vi "IMU_read_RT_streaming_data_1.0.vi"() -> ()   [LabVIEW 2016]
doc: "This example demonstrates how to stream data from the FPGA target to the host PC using DMA FIFO."
uses:
  <vilib>/userdefined/Silver/nirio_resource_slv.ctl
  <vilib>/FPGAPlugInAG/cRIO-9116/niLvFpga_Open_cRIO-9116.vi
  <vilib>/rvi/interface/common/dynamic/niFpgaDynamicAddResources.vi
  <vilib>/Utility/error.llb/Error Cluster From Error Code.vi
  <vilib>/rvi/errors/niLvFpgaAdjustHostInterfaceError.vi
  <vilib>/FPGAPlugInAG/Dynamic/niLvFpga_Close_Dynamic.vi
  <vilib>/rvi/interface/nirviOpenFPGA/nirviOpenFPGA.xnode
  FPGA Bitfiles/IMUuse_FPGATarget_IMUreadFPGAstrea_DORLY4QJmyg.lvbitx
  IMU_read_FPGA_streaming_data.vi
  <vilib>/rvi/interface/nirviReadWriteControl/nirviReadWriteControl.xnode
  <vilib>/rvi/interface/nirviMethod/nirviMethod.xnode
  <vilib>/rvi/interface/nirviCloseFPGA/nirviCloseFPGA.xnode
  <vilib>/FPGAPlugInAG/Dynamic/niLvFpga_ReadFifo_Dynamic.vi
  <vilib>/rvi/errors/niLvFpgaMergeErrorWithErrorCode.vi
  NiFpgaLv.dll
  <vilib>/rvi/interface/Simulation/niFpgaSimulationCallBeginRW.vi
panel:
  out "Angle (degree)":cluster{ext, ext, ext}(graph)
  out "Angular Rate (degree/s)":cluster{ext, ext, ext}(graph)
  in  "停止按钮":bool
  in  "波特率":T1(ring)=enum."460.8 kbps"
  in  "RIO Device":T2="RIO0"
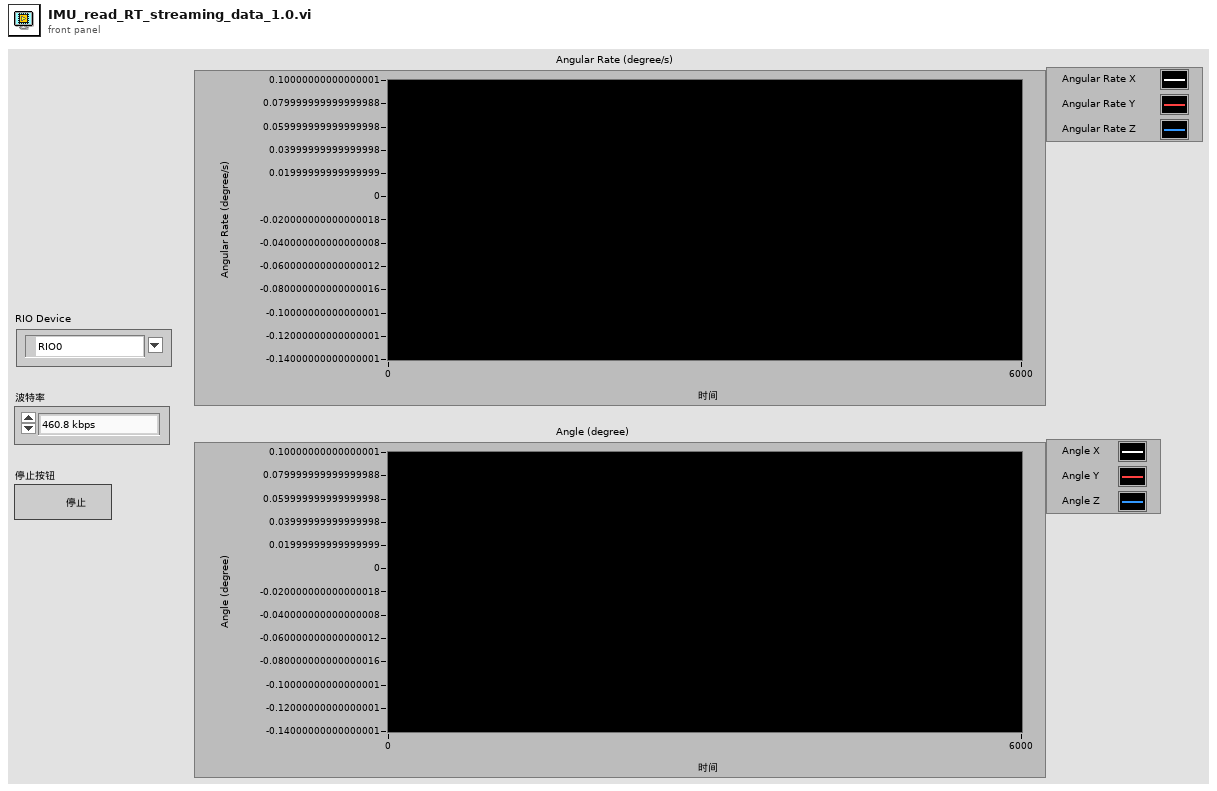
[diagram p1: front panel]
types:
  T1 = enum16{"75 bps", "110 bps", "134 bps", "150 bps", "300 bps", "600 bps", "1200 bps", "1800 bps", "2400 bps", "4800 bps", "7200 bps", "9600 bps", "14.4 kbps", "19.2 kbps", "28.8 kbps", "38.4 kbps", "57.6 kbps", "115.2 kbps", "230.4 kbps", "460.8 kbps", "921.6 kbps"}
  T2 = typedef "nirio_resource_slv.ctl" = tag
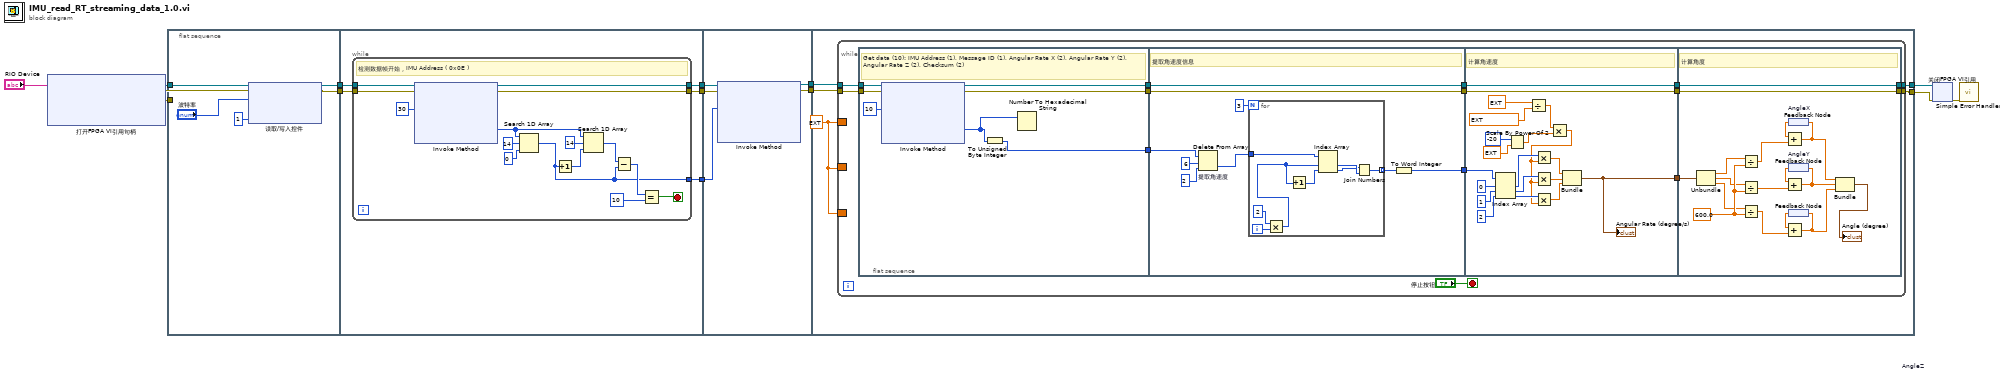
[diagram p0: block diagram]
diagram:
  n1 = xnode "打开FPGA VI引用句柄"("资源名称"="RIO Device") -> ("FPGA VI引用输出"=w12:refnum<k20>, "错误输出"=w11:errorcluster)  [unwired: 1 in]
  n2 = flat-sequence {
    tunnel: w12 -> [w19]
    tunnel: w11 -> [w18]
    tunnel: [w17] -> w9
    tunnel: [w16] -> w8
    tunnel: w9 -> [w24]
    tunnel: w8 -> [w23]
    tunnel: [w22] -> w7
    tunnel: [w21] -> w6
    tunnel: [w20] -> w5
    tunnel: w7 -> [w44]
    tunnel: w6 -> [w43]
    tunnel: w5 -> [w42]
    tunnel: [w41] -> w4
    tunnel: [w40] -> w3
    tunnel: w4 -> [w49]
    tunnel: w3 -> [w48]
    tunnel: [w47] -> w2
    tunnel: [w46] -> w1
    frame #0 {
      n3 = xnode "读取/写入控件"("FPGA VI引用输入"=w19, "错误输入"=w18, "波特率"="波特率", "Number of bytes"=u16 1) -> ("FPGA VI引用输出"=w17:refnum<k20>, "错误输出"=w16:errorcluster)  [unwired: 1 out]
    }
    frame #1 {
      n4 = while "While循环" {
        tunnel: w23 -> [w38]
        tunnel: [w36] -> w21
        tunnel: w24 -> [w39]
        tunnel: [w37] -> w22
        tunnel: [w25] -> w20
        stop <- w26 stop-if-true
        # "检测数据帧开始，IMU Address ( 0x0E )"
        n5 = xnode "Invoke Method"("FPGA VI引用输入"=w39, "错误输入"=w38, "元素数量"=u32 30) -> ("FPGA VI引用输出"=w37:refnum<k20>, "错误输出"=w36:errorcluster, "数据"=w31:i16[])  [unwired: 1 in, 1 out]
        n6 = Search 1D Array(1D array=w31, element=i16 14 ("IMU Address"), start index (0)=0 ("开始索引(0)")) -> (index of element=w25:i32)
        n7 = Increment(x=w25) -> (x+1=w33:i32)
        n8 = Search 1D Array(1D array=w31, element=i16 14 ("IMU Address"), start index (0)=w33) -> (index of element=w32:i32)
        n9 = Subtract(x=w32, y=w25) -> (x-y=w29:i32)
        n10 = Equal?(x=w29, y=10) -> (x = y?=w26:bool)
      }
    }
    frame #2 {
      n11 = xnode "Invoke Method"("FPGA VI引用输入"=w44, "错误输入"=w43, "元素数量"=w42) -> ("FPGA VI引用输出"=w41:refnum<k20>, "错误输出"=w40:errorcluster)  [unwired: 1 in, 2 out]
    }
    frame #3 {
      w45 = ext 0.0
      n12 = while {
        tunnel: w48 -> [w62]
        tunnel: [w60] -> w46
        tunnel: w49 -> [w63]
        tunnel: [w61] -> w47
        border: w45 -> [_]
        border: w45 -> [_]
        border: w45 -> [_]
        stop <- "停止按钮" stop-if-true
        n13 = flat-sequence "平铺式顺序结构" {
          tunnel: w63 -> [w70]
          tunnel: w62 -> [w69]
          tunnel: [w68] -> w58
          tunnel: [w67] -> w57
          tunnel: [w64] -> w56
          tunnel: w58 -> [w79]
          tunnel: w57 -> [w78]
          tunnel: w56 -> [w73]
          tunnel: [w79] -> w55
          tunnel: [w78] -> w54
          tunnel: [w71] -> w53
          tunnel: w55 -> [w107]
          tunnel: w54 -> [w106]
          tunnel: w53 -> [w98]
          tunnel: [w107] -> w52
          tunnel: [w106] -> w51
          tunnel: [w88] -> w50
          tunnel: [w123] -> w60
          tunnel: [w124] -> w61
          tunnel: w52 -> [w124]
          tunnel: w51 -> [w123]
          tunnel: w50 -> [w122]
          frame #0 {
            # "Get data (10): IMU Address (1), Message ID (1), Angular Rate X (2), Angular Rate Y (2), Angular Rate Z (2), Checksum (2)"
            n14 = xnode "Invoke Method"("FPGA VI引用输入"=w70, "错误输入"=w69, "元素数量"=u32 10) -> ("FPGA VI引用输出"=w68:refnum<k20>, "错误输出"=w67:errorcluster, "数据"=w65:i16[])  [unwired: 1 in, 1 out]
            n15 = To Unsigned Byte Integer(number=w65) -> (unsigned 8bit integer=w64:u8[])
            n16 = Number To Hexadecimal String(2:w65) -> ()  [unwired: 1 in, 1 out]
          }
          frame #1 {
            # "提取角速度信息"
            n17 = Delete From Array "提取角速度"(array=w73, length=6 ("数据域长度"), index=2 ("角速度数据开始位置")) -> (deleted portion=w74:u8[])  [unwired: 1 out]
            n18 = for {
              N: 3 -> [_]
              tunnel: w74 -> [w84]
              tunnel: [w81] -> w72 mode=indexing
              i -> [w87]
              n19 = Multiply(x=2, y=w87) -> (x*y=w80:i32)
              n20 = Increment(x=w80) -> (x+1=w85:i32)
              n21 = Index Array(array=w84, index #1=w80, index #2=w85) -> (element #1=w83:u8, element #2=w82:u8)
              n22 = Join Numbers(hi=w82, lo=w83) -> ((hi.lo)=w81:u16)
            }
            n23 = To Word Integer(number=w72) -> (16bit integer=w71:i16[])
          }
          frame #2 {
            # "计算角速度"
            n24 = Index Array(array=w98, index #1=0 ("索引"), index #2=1 ("索引"), index #3=2 ("索引")) -> (element #1=w96:i16, element #2=w95:i16, element #3=w97:i16)
            n25 = Scale By Power Of 2 ("按2的幂缩放")(n=i16 -20, x=ext 600.0) -> (x*2^n=w91:ext)
            n26 = Divide(x=ext 180.0 ("y"), y=ext 3.141592653) -> (x/y=w92:ext)
            n27 = Multiply(x=w92, y=w91) -> (x*y=w90:ext)
            n28 = Multiply(x=w96, y=w90) -> (x*y=w105:ext)
            n29 = Multiply(x=w95, y=w90) -> (x*y=w104:ext)
            n30 = Multiply(x=w97, y=w90) -> (x*y=w89:ext)
            n31 = Bundle(w105, w104, w89) -> (w88:cluster{ext, ext, ext})  [unwired: 1 in]
            "Angular Rate (degree/s)" <- w88
          }
          frame #3 {
            w121 = 600.0 ("数据频率")
            # "计算角度"
            n32 = Unbundle(w122) -> (w118:ext, w119:ext, w120:ext)
            n33 = Divide(x=w118, y=w121) -> (x/y=w114:ext)
            n34 = Divide(x=w119, y=w121) -> (x/y=w115:ext)
            n35 = Divide(x=w120, y=w121) -> (x/y=w116:ext)
            n36 = feedback #1 "AngleX"() -> (w112:ext)
            n37 = Add(x=w112, y=w114) -> (x+y=w110:ext)
            n38 = feedback-in #1(w110) -> ()
            n39 = feedback #2 "AngleY"() -> (w113:ext)
            n40 = Add(x=w113, y=w115) -> (x+y=w111:ext)
            n41 = feedback-in #2(w111) -> ()
            n42 = feedback #3 "AngleZ"() -> (w117:ext)
            n43 = Add(x=w117, y=w116) -> (x+y=w109:ext)
            n44 = feedback-in #3(w109) -> ()
            n45 = Bundle(w110, w111, w109) -> (→"Angle (degree)":cluster{ext, ext, ext})  [unwired: 1 in]
          }
        }
      }
    }
  }
  n46 = xnode "关闭FPGA VI引用"("FPGA VI引用输入"=w2, "错误输入"=w1) -> ("错误输出"=w10:errorcluster)
  n47 = call <vilib>:"Simple Error Handler.vi"("error in (no error)"=w10) -> ()  [unwired: 4 in, 5 out]
